vi "BartlomiejLechman_prac9_2.vi"() -> ()   [LabVIEW 2019]
uses:
  <vilib>/Platform/TimedLoop/XDataNode/timing_clust.ctl
  <vilib>/Platform/TimedLoop/XDataNode/nitl_modes.ctl
  <vilib>/Platform/TimedLoop/XDataNode/wakeup.ctl
  <vilib>/platform/TimedLoop/XDataNode/XDataNode.xnode
  <vilib>/Platform/TimedLoop/XDataNode/XDNodeRunTimeDep.lvlib
panel:
  out "error out":errorcluster
  out "Waveform Graph":waveform(dbl)(graph)
  in  "stop":bool
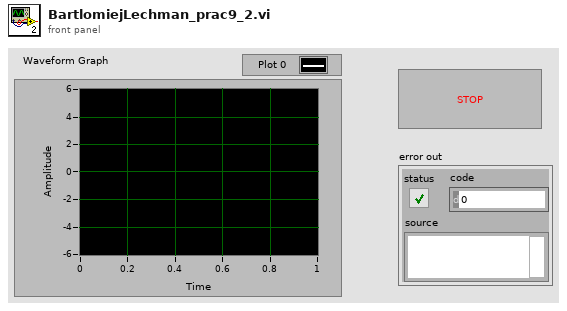
[diagram p1: front panel]
types:
  T1 = typedef "XDNodeRunTimeDep.lvlib/timing_clust.ctl" = cluster{"Expected End [f-1]":u64, "Actual End [f-1]":u64, "Finished Late? [f-1]":bool, "Expected End [i-1]":u64, "Actual End [i-1]":u64, "Finished Late? [i-1]":bool, "Expected Start [i]":u64, "Actual Start [i]":u64, "Expected Start [f]":u64, "Actual Start [f]":u64, "Source Name":string, "Structure Name":string, "Period":i64, "Deadline":i64, "Offset":i64, "Start":i64, "Priority":i32, "Timeout":i32, "Mode":T2, "Wakeup Reason":T3, "Error":errorcluster, "Source Type":string, "Secondary Source Type":string, "Global End Time":u64, "Global Start Time":u64, "Frame Duration":u64, "Iteration Duration":u64, "Assigned CPU":i32, "I/O Scan Engine Mode":u32}
  T2 = typedef "XDNodeRunTimeDep.lvlib/nitl_modes.ctl" = enum32{"No Change", "Process missed periods, maintain original phase", "Discard missed periods, maintain original phase", "Process missed periods, ignore original phase", "Discard missed periods, ignore original phase"}
  T3 = typedef "XDNodeRunTimeDep.lvlib/wakeup.ctl" = enum32{"Normal", "Aborted", "Asynchronous wakeup", "Timing source error", "Timed loop error", "Timeout"}
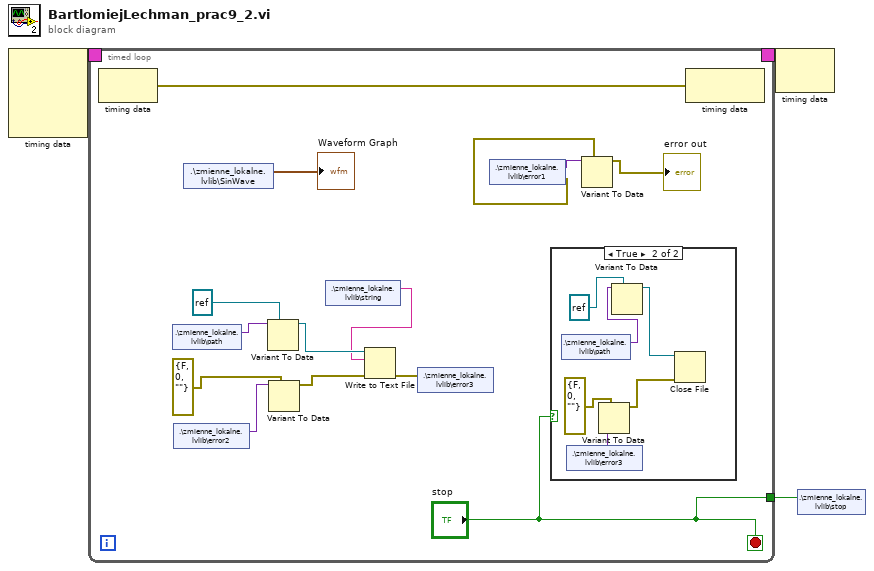
[diagram p0: block diagram]
diagram:
  n1 = node-c288() -> (w3:T1)  [unwired: 4 in]
  n2 = timed-loop {
    timing: w3 -> [_]
    timing-out: [_] -> w2
    tunnel: ["stop"] -> w1
    stop <- "stop" stop-if-true
    n3 = node-c288() -> (w13:errorcluster)  [unwired: 1 in]
    n4 = shared-variable ".\\zmienne_lokalne.lvlib\\path"() -> (w11:variant)  [unwired: 1 in, 1 out]
    n5 = shared-variable ".\\zmienne_lokalne.lvlib\\error2"() -> (w8:variant)  [unwired: 1 in, 1 out]
    n6 = shared-variable ".\\zmienne_lokalne.lvlib\\SinWave"() -> (→"Waveform Graph":waveform(dbl))  [unwired: 1 in, 1 out]
    n7 = Variant To Data(type=refnum<file> refnum ("refnum out"), Variant=w11) -> (data=w7:refnum<file>)  [unwired: 1 in, 1 out]
    n8 = Variant To Data(type=errorcluster {"status"=FALSE, "code"=0, "source"=""} ("error out"), Variant=w8) -> (data=w6:errorcluster)  [unwired: 1 in, 1 out]
    n9 = shared-variable ".\\zmienne_lokalne.lvlib\\string"() -> (w5:string)  [unwired: 1 in, 1 out]
    n10 = Write to Text File(file (use dialog)=w7, text=w5, error in=w6) -> (error out=w4:errorcluster)  [unwired: 1 in, 2 out]
    n11 = shared-variable ".\\zmienne_lokalne.lvlib\\error3"(w4) -> ()  [unwired: 1 in, 1 out]
    n12 = shared-variable ".\\zmienne_lokalne.lvlib\\error1"() -> (w16:variant, error out=w14:errorcluster)  [unwired: 1 in]
    n13 = case shown="True" "stop" {
      frame False {
      }
      frame True {
        n14 = shared-variable ".\\zmienne_lokalne.lvlib\\path"() -> (w20:variant)  [unwired: 1 in, 1 out]
        n15 = shared-variable ".\\zmienne_lokalne.lvlib\\error3"() -> (w23:variant)  [unwired: 1 in, 1 out]
        n16 = Variant To Data(type=errorcluster {"status"=FALSE, "code"=0, "source"=""} ("error out"), Variant=w23) -> (data=w21:errorcluster)  [unwired: 1 in, 1 out]
        n17 = Variant To Data(type=refnum<file> refnum ("refnum out"), Variant=w20) -> (data=w18:refnum<file>)  [unwired: 1 in, 1 out]
        n18 = Close File(refnum=w18, error in=w21) -> ()  [unwired: 2 out]
      }
    }
    n19 = Variant To Data(type=w14, Variant=w16) -> (data=→"error out":errorcluster)  [unwired: 1 in, 1 out]
    n20 = node-c288(w13) -> ()  [unwired: 1 out]
  }
  n21 = node-c288(w2) -> ()  [unwired: 1 out]
  n22 = shared-variable ".\\zmienne_lokalne.lvlib\\stop"(w1) -> ()  [unwired: 1 in, 1 out]
